vi "DynamicConstantCurrScan.vi"() -> ()   [LabVIEW 2014]
uses:
  <vilib>/userdefined/High Color/nirio_resource_hc.ctl
  <vilib>/Instr/_visa.llb/VISA Configure Serial Port (Instr).vi
  <vilib>/FPGAPlugInAG/PCIe-7851R/niLvFpga_Open_PCIe-7851R.vi
  <vilib>/rvi/interface/common/dynamic/niFpgaDynamicAddResources.vi
  <vilib>/Utility/error.llb/Error Cluster From Error Code.vi
  <vilib>/rvi/errors/niLvFpgaAdjustHostInterfaceError.vi
  <vilib>/FPGAPlugInAG/Dynamic/niLvFpga_Close_Dynamic.vi
  <vilib>/rvi/interface/nirviOpenFPGA/nirviOpenFPGA.xnode
  FPGA Bitfiles/FPGATest_FPGATarget_PIZApproaching_ngy2QjQf4ns.lvbitx
  <vilib>/rvi/interface/nirviReadWriteControl/nirviReadWriteControl.xnode
  <vilib>/rvi/interface/nirviCloseFPGA/nirviCloseFPGA.xnode
  FPGA Bitfiles/FPGATest_FPGATarget_ProbeAdjustment_Nyu9RVmYDZg.lvbitx
  FPGA Bitfiles/FPGATest_FPGATarget_PIZWithdraw_LXoQbY-wYvI.lvbitx
  NiFpgaLv.dll
  <vilib>/rvi/interface/Simulation/niFpgaSimulationCallBeginRW.vi
  NextXYPos.dll
panel:
  in  "zRisingLimitLen / um":dbl format="%#_13g"
  in  "ScanStop":bool
  out "refCurrIndex":i32
  out "preCurrIndexDia":i16(graph)
  out "ZPosDia":i16(graph)
  out "PIZPosIndex":i32
  out "preCurrIndex":i32
  in  "ApproachStop":bool
  out "ThresholdLowerBound":i32
  out "ThresholdUpperBound":i32
  in  "DeclineTolerantInterval %":dbl format="%#_13g"
  in  "AdjustStepMultiplier/0.305nm":i32
  in  "ApproachStepMultiplier/0.305nm":i32
  in  "PIZ":T1
  in  "ProbeBrokenIndex":i32
  in  "ThresholdIndex":i32
  in  "ScanNumToRefresh":i32
  out "YPos?":dbl
  out "XPos?":dbl
  in  "YInitStepLen / um":dbl format="%#_13g"
  in  "XInitStepLen / um":dbl format="%#_13g"
  in  "YDirTotalLen / um":dbl format="%#_13g"
  in  "XDirTotalLen / um":dbl format="%#_13g"
  in  "Y Init / um":dbl format="%#_13g"
  in  "X Init / um":dbl format="%#_13g"
  out "RoughXYZErr?":string
  in  "RoughXYZ":refnum<visa-resource-name>
  in  "AllLoopSleep ms":i32
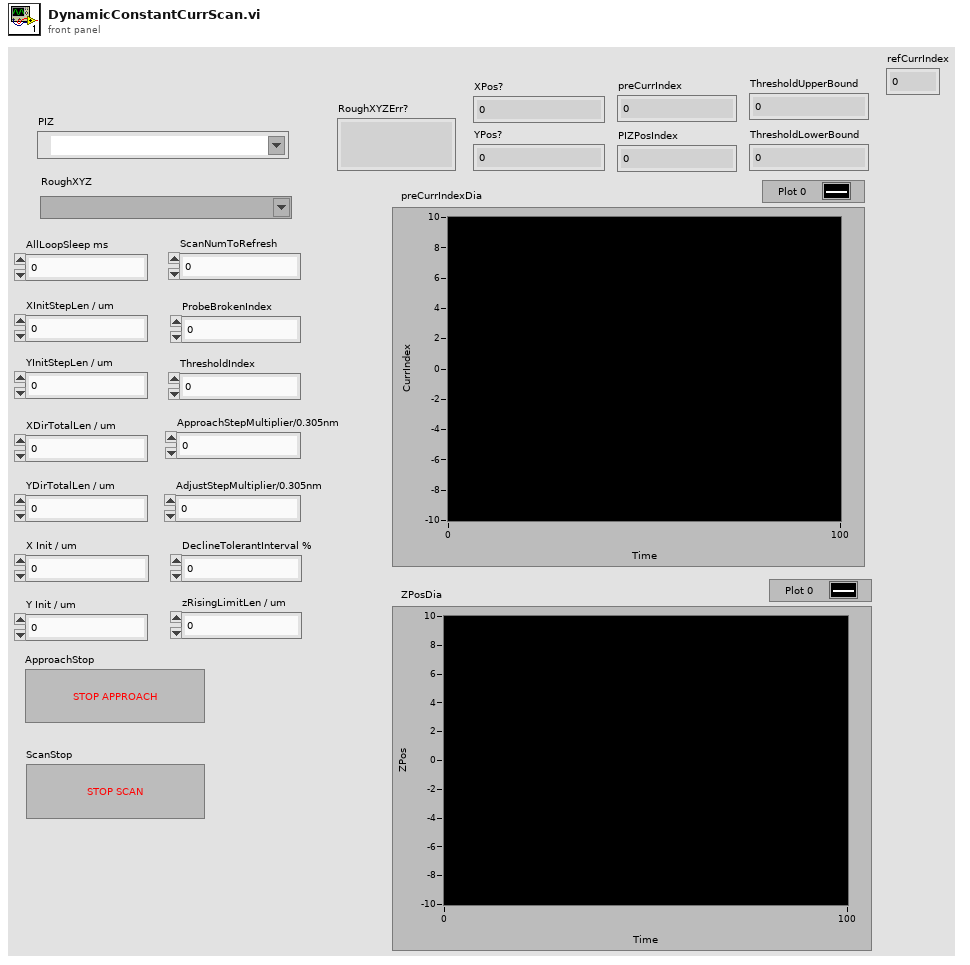
[diagram p1: front panel]
types:
  T1 = typedef "nirio_resource_hc.ctl" = tag
diagram:
  n1 = flat-sequence {
    tunnel: [w69] -> w52
    tunnel: [w68] -> w51
    tunnel: w52 -> [w111]
    tunnel: w51 -> [w110]
    tunnel: [w95] -> w50
    tunnel: [w94] -> w49
    tunnel: w50 -> [w113]
    tunnel: w49 -> [w112]
    tunnel: [w113] -> w48
    tunnel: [w112] -> w47
    tunnel: w48 -> [w118]
    tunnel: w47 -> [w117]
    tunnel: [w116] -> w46
    tunnel: [w115] -> w44
    tunnel: w46 -> [w144]
    tunnel: [w144] -> w45
    tunnel: w44 -> [w143]
    tunnel: [w143] -> w43
    tunnel: [w139] -> w42
    tunnel: [w138] -> w41
    tunnel: [w135] -> w40
    tunnel: w45 -> [w151]
    tunnel: w43 -> [w150]
    tunnel: w42 -> [w153]
    tunnel: w41 -> [w152]
    tunnel: w40 -> [w149]
    tunnel: [w146] -> w39
    tunnel: [w145] -> w38
    tunnel: w39 -> [w220]
    tunnel: w38 -> [w219]
    tunnel: [w220] -> w37
    tunnel: [w219] -> w36
    tunnel: [w214] -> w35
    tunnel: [w213] -> w34
    tunnel: [w213] -> w33
    tunnel: [1] -> w32
    tunnel: [w211] -> w31
    tunnel: [w210] -> w30
    tunnel: [w209] -> w29
    tunnel: [w208] -> w28
    tunnel: [0] -> w27
    tunnel: [w206] -> w26
    tunnel: [w206] -> w25
    tunnel: [w206] -> w24
    tunnel: [w206] -> w23
    tunnel: [i32[] []] -> w22
    tunnel: [w193] -> w21
    tunnel: [w192] -> w20
    tunnel: w37 -> [w248]
    tunnel: w36 -> [w247]
    tunnel: w35 -> [w246]
    tunnel: w34 -> [w237]
    tunnel: w33 -> [w236]
    tunnel: w32 -> [w240]
    tunnel: w31 -> [w239]
    tunnel: w30 -> [w238]
    tunnel: w29 -> [w242]
    tunnel: w28 -> [w241]
    tunnel: w27 -> [w243]
    tunnel: w26 -> [w230]
    tunnel: w25 -> [w229]
    tunnel: w24 -> [w228]
    tunnel: w23 -> [w227]
    tunnel: w22 -> [w226]
    tunnel: w21 -> [w245]
    tunnel: w20 -> [w244]
    tunnel: [w235] -> w19
    tunnel: [w234] -> w18
    tunnel: [w233] -> w17
    tunnel: [w232] -> w16
    tunnel: [w231] -> w15
    tunnel: [w225] -> w14
    tunnel: [w224] -> w13
    tunnel: [w223] -> w12
    tunnel: [w222] -> w11
    tunnel: w19 -> [_]
    tunnel: w18 -> [_]
    tunnel: w17 -> [_]
    tunnel: w16 -> [_]
    tunnel: w15 -> [_]
    tunnel: w14 -> [w863]
    tunnel: w13 -> [w861]
    tunnel: w12 -> [w860]
    tunnel: w11 -> [w862]
    tunnel: [w857] -> w10
    tunnel: [w856] -> w9
    tunnel: [w851] -> w8
    tunnel: [w850] -> w7
    tunnel: w10 -> [w869]
    tunnel: w9 -> [w868]
    tunnel: w8 -> [w871]
    tunnel: w7 -> [w870]
    tunnel: [w867] -> w6
    tunnel: [w866] -> w5
    tunnel: [w865] -> w4
    tunnel: [w864] -> w3
    tunnel: w6 -> [w906]
    tunnel: w5 -> [w905]
    tunnel: w4 -> [w904]
    tunnel: w3 -> [w903]
    tunnel: [w902] -> w2
    tunnel: [w901] -> w1
    tunnel: w2 -> [w915]
    tunnel: w1 -> [w914]
    frame #0 {
      n2 = call-poly "VISA Configure Serial Port"("VISA resource name"="RoughXYZ", "baud rate (9600)"=u32 115200) -> ("VISA resource name out"=w78:refnum<visa-resource-name>, "error out"=w77:errorcluster)  [unwired: 12 in]
      n3 = local write "DeclineTolerantInterval %"("DeclineTolerantInterval %") -> ()
      n4 = local write "AllLoopSleep ms"("AllLoopSleep ms") -> ()
      n5 = local write "XDirTotalLen / um"("XDirTotalLen / um") -> ()
      n6 = local write "YDirTotalLen / um"("YDirTotalLen / um") -> ()
      n7 = local write "XInitStepLen / um"("XInitStepLen / um") -> ()
      n8 = local write "YInitStepLen / um"("YInitStepLen / um") -> ()
      n9 = local write "zRisingLimitLen / um"("zRisingLimitLen / um") -> ()
      n10 = local write "X Init / um"("X Init / um") -> ()
      n11 = local write "Y Init / um"("Y Init / um") -> ()
      n12 = local write "PIZ"("PIZ") -> ()
      n13 = VISA Write(VISA resource name=w78, write buffer="ERR?\n", error in (no error)=w77) -> (VISA resource name out=w75:refnum<visa-resource-name>, error out=w74:errorcluster)  [unwired: 1 out]
      n14 = VISA Read(VISA resource name=w75, byte count=u32 128, error in (no error)=w74) -> (VISA resource name out=w72:refnum<visa-resource-name>, read buffer=→"RoughXYZErr?":string, error out=w71:errorcluster)  [unwired: 1 out]
      n15 = local write "ProbeBrokenIndex"("ProbeBrokenIndex") -> ()
      n16 = local write "ScanNumToRefresh"("ScanNumToRefresh") -> ()
      n17 = local write "ApproachStepMultiplier/0.305nm"("ApproachStepMultiplier/0.305nm") -> ()
      n18 = local write "ThresholdIndex"("ThresholdIndex") -> ()
      n19 = local write "AdjustStepMultiplier/0.305nm"("AdjustStepMultiplier/0.305nm") -> ()
      n20 = VISA Write(VISA resource name=w72, write buffer="ONL 1 1 2 1 3 1\nSVO A 1\nSVO B 1\nSVO C 1\nMOV A 0\nMOV B 0\n", error in (no error)=w71) -> (VISA resource name out=w69:refnum<visa-resource-name>, error out=w68:errorcluster)  [unwired: 1 out]
    }
    frame #1 {
      n21 = local read "DeclineTolerantInterval %"() -> (w92:dbl)
      n22 = local read "ThresholdIndex"() -> (w89:i32)
      n23 = local read "X Init / um"() -> (w107:dbl)
      n24 = Number To Fractional String(number=w107, precision (6)=i16 10) -> (F-format string=w105:string)  [unwired: 2 in]
      n25 = Concatenate Strings("MOV A " ("string"), w105, "\n" ("string")) -> (w102:string)
      n26 = Divide(x=w92, y=100.0) -> (x/y=w90:dbl)
      n27 = VISA Write(VISA resource name=w111, write buffer=w102, error in (no error)=w110) -> (VISA resource name out=w109:refnum<visa-resource-name>, error out=w108:errorcluster)  [unwired: 1 out]
      n28 = Multiply(x=w89, y=w90) -> (x*y=w88:dbl)
      n29 = local read "Y Init / um"() -> (w101:dbl)
      n30 = Add(x=w89, y=w88) -> (x+y=w87:dbl)
      n31 = Subtract(x=w89, y=w88) -> (x-y=w86:dbl)
      n32 = Round Toward +Infinity(x=w87) -> (ceil(x): smallest int >= x=w85:dbl)
      n33 = Wait (ms)(milliseconds to wait=u32 200) -> ()  [unwired: 1 out]
      n34 = Round Toward -Infinity(1:w86) -> (0:w84:dbl)
      n35 = To Long Integer(number=w85) -> (32bit integer=→"ThresholdUpperBound":i32)
      n36 = To Long Integer(number=w84) -> (32bit integer=→"ThresholdLowerBound":i32)
      n37 = Number To Fractional String(number=w101, precision (6)=i16 10) -> (F-format string=w98:string)  [unwired: 2 in]
      n38 = Concatenate Strings("MOV B " ("string"), w98, "\n" ("string")) -> (w96:string)
      n39 = VISA Write(VISA resource name=w109, write buffer=w96, error in (no error)=w108) -> (VISA resource name out=w95:refnum<visa-resource-name>, error out=w94:errorcluster)  [unwired: 1 out]
    }
    frame #2 {
      n40 = Wait (ms)(milliseconds to wait=u32 1500) -> ()  [unwired: 1 out]
    }
    frame #3 {
      n41 = VISA Write(VISA resource name=w118, write buffer="POS? A\n", error in (no error)=w117) -> (VISA resource name out=w133:refnum<visa-resource-name>, error out=w132:errorcluster)  [unwired: 1 out]
      n42 = VISA Read(VISA resource name=w133, byte count=u32 128, error in (no error)=w132) -> (VISA resource name out=w127:refnum<visa-resource-name>, read buffer=w124:string, error out=w126:errorcluster)  [unwired: 1 out]
      n43 = Fract/Exp String To Number(string=w124, offset=2) -> (number=→"XPos?":dbl)  [unwired: 2 in, 1 out]
      n44 = VISA Write(VISA resource name=w127, write buffer="POS? B\n", error in (no error)=w126) -> (VISA resource name out=w130:refnum<visa-resource-name>, error out=w129:errorcluster)  [unwired: 1 out]
      n45 = VISA Read(VISA resource name=w130, byte count=u32 128, error in (no error)=w129) -> (VISA resource name out=w116:refnum<visa-resource-name>, read buffer=w119:string, error out=w115:errorcluster)  [unwired: 1 out]
      n46 = Fract/Exp String To Number(string=w119, offset=2) -> (number=→"YPos?":dbl)  [unwired: 2 in, 1 out]
    }
    frame #4 {
      n47 = local read "PIZ"() -> (w142:T1)
      n48 = xnode "Open FPGA VI Reference"("resource name"=w142) -> ("FPGA VI Reference Out"=w141:refnum<k20>, "error out"=w140:errorcluster)  [unwired: 1 in]
      n49 = local read "ApproachStepMultiplier/0.305nm"() -> (w136:i32)
      n50 = local read "AllLoopSleep ms"() -> (w135:i32)
      n51 = local read "ThresholdIndex"() -> (w137:i32)
      n52 = xnode "Read/Write Control"("FPGA VI Reference In"=w141, "error in"=w140, "Sleep ms"=w135, "thresholdIndex"=w137, "stepMultiplier / 0.305nm"=w136) -> ("FPGA VI Reference Out"=w139:refnum<k20>, "error out"=w138:errorcluster)
    }
    frame #5 {
      n53 = while {
        tunnel: w153 -> [w172]
        tunnel: w152 -> [w171]
        tunnel: w151 -> [w166]
        tunnel: w150 -> [w164]
        tunnel: w149 -> [w160]
        tunnel: [w157] -> w148
        tunnel: [w156] -> w147
        tunnel: [w155] -> w146
        tunnel: [w154] -> w145
        stop <- w163 stop-if-true
        n54 = flat-sequence {
          tunnel: w172 -> [w184]
          tunnel: w171 -> [w183]
          tunnel: [w182] -> w170
          tunnel: [w181] -> w169
          tunnel: ["ApproachStop"] -> w168
          tunnel: [w179] -> w167
          tunnel: w166 -> [w179]
          tunnel: [w178] -> w165
          tunnel: w164 -> [w178]
          tunnel: [w177] -> w161
          tunnel: w160 -> [w177]
          tunnel: [w176] -> w159
          tunnel: w170 -> [w186]
          tunnel: w169 -> [w185]
          tunnel: [w191] -> w162
          tunnel: w168 -> [w191]
          tunnel: [w190] -> w155
          tunnel: w167 -> [w190]
          tunnel: w165 -> [w189]
          tunnel: [w189] -> w154
          tunnel: w161 -> [w188]
          tunnel: w159 -> [w187]
          tunnel: [w187] -> w158
          tunnel: [w186] -> w157
          tunnel: [w185] -> w156
          frame #0 {
            n55 = xnode "Read/Write Control"("FPGA VI Reference In"=w184, "error in"=w183, "stop"="ApproachStop") -> ("FPGA VI Reference Out"=w182:refnum<k20>, "error out"=w181:errorcluster, "preCurrIndex"=→"preCurrIndex" →"preCurrIndexDia":i16, "PIZPos"=→"PIZPosIndex" →"ZPosDia":i16, "Approached?"=w176:bool, "refCurrIndex"=→"refCurrIndex":i16)
          }
          frame #1 {
            n56 = Wait (ms)(milliseconds to wait=w188) -> ()  [unwired: 1 out]
          }
        }
        n57 = Or(x=w158, y=w162) -> (x .or. y?=w163:bool)
      }
      n58 = xnode "Close FPGA VI Reference"("FPGA VI Reference In"=w148, "error in"=w147) -> ()  [unwired: 1 out]
    }
    frame #6 {
      w206 = dbl[] []
      w213 = 0
      # "zPosIndex"
      # "yReal"
      # "yCal"
      # "xReal"
      # "xCal"
      # "LastZPos"
      # "yCalPos"
      # "xCalPos"
      # "yStepLen"
      # "xStepLen"
      # "xVel"
      # "yCounting"
      # "xCounting"
      # "xPreviousNum"
      n59 = local read "PIZ"() -> (w204:T1)
      n60 = local read "XDirTotalLen / um"() -> (w218:dbl)
      n61 = local read "XInitStepLen / um"() -> (w217:dbl)
      n62 = Wait (ms)(milliseconds to wait=u32 50) -> ()  [unwired: 1 out]
      n63 = xnode "Open FPGA VI Reference"("resource name"=w204) -> ("FPGA VI Reference Out"=w203:refnum<k20>, "error out"=w202:errorcluster)  [unwired: 1 in]
      n64 = local read "AdjustStepMultiplier/0.305nm"() -> (w196:i32)
      n65 = local read "ThresholdUpperBound"() -> (w201:i32)
      n66 = local read "ThresholdLowerBound"() -> (w200:i32)
      n67 = local read "ScanNumToRefresh"() -> (w197:i32)
      n68 = local read "ProbeBrokenIndex"() -> (w198:i32)
      n69 = local read "AllLoopSleep ms"() -> (w194:i32)
      n70 = local read "ThresholdIndex"() -> (w199:i32)
      n71 = local read "refCurrIndex"() -> (w195:i32)
      n72 = Divide(x=w218, y=w217) -> (x/y=w216:dbl)
      n73 = Round Toward +Infinity(x=w216) -> (ceil(x): smallest int >= x=w215:dbl)
      n74 = To Long Integer(number=w215) -> (32bit integer=w214:i32)
      n75 = xnode "Read/Write Control"("FPGA VI Reference In"=w203, "error in"=w202, "ThresholdUpperBound"=w201, "ThresholdLowerBound"=w200, "ThresholdIndex"=w199, "ProbeBrokenIndex"=w198, "ScanNumToRefresh"=w197, "stepMultiplier/0.305nm"=w196, "refCurrIndex"=w195, "Sleep ms"=w194) -> ("FPGA VI Reference Out"=w193:refnum<k20>, "error out"=w192:errorcluster)
      n76 = local read "XInitStepLen / um"() -> (w211:dbl)
      n77 = local read "YInitStepLen / um"() -> (w210:dbl)
      n78 = local read "X Init / um"() -> (w209:dbl)
      n79 = local read "Y Init / um"() -> (w208:dbl)
    }
    frame #7 {
      n80 = while {
        tunnel: w248 -> [w405]
        tunnel: w247 -> [w404]
        tunnel: w246 -> [w365]
        tunnel: w245 -> [w393]
        tunnel: w244 -> [w392]
        shift-right: [w285] -> _
        shift-left: w237 -> [w274]
        shift-right: [w284] -> _
        shift-left: w236 -> [w273]
        shift-right: [w283] -> _
        shift-left: w240 -> [w277]
        shift-right: [w281] -> _
        shift-left: w239 -> [w276]
        shift-right: [w282] -> _
        shift-left: w238 -> [w275]
        shift-right: [w288] -> _
        shift-left: w242 -> [w279]
        shift-right: [w287] -> _
        shift-left: w241 -> [w278]
        shift-right: [w286] -> _
        shift-left: w243 -> [w280]
        shift-right: [w272] -> w235
        shift-left: w230 -> [w267]
        shift-right: [w271] -> w234
        shift-left: w229 -> [w266]
        shift-right: [w270] -> w233
        shift-left: w228 -> [w265]
        shift-right: [w269] -> w232
        shift-left: w227 -> [w264]
        shift-right: [w268] -> w231
        shift-left: w226 -> [w263]
        tunnel: [w262] -> w224
        tunnel: [w261] -> w223
        tunnel: [w258] -> w225
        tunnel: [w257] -> w222
        stop <- w253 stop-if-true
        n81 = flat-sequence {
          tunnel: w405 -> [w441]
          tunnel: w404 -> [w440]
          tunnel: [w429] -> w403
          tunnel: [w428] -> w402
          tunnel: [w421] -> w401
          tunnel: w279 -> [w421]
          tunnel: [w420] -> w400
          tunnel: w278 -> [w420]
          tunnel: [w419] -> w399
          tunnel: w280 -> [w419]
          tunnel: w393 -> [w418]
          tunnel: w392 -> [w417]
          tunnel: [w418] -> w389
          tunnel: [w417] -> w386
          tunnel: [w416] -> w380
          tunnel: w267 -> [w416]
          tunnel: [w415] -> w379
          tunnel: w266 -> [w415]
          tunnel: [w414] -> w378
          tunnel: w265 -> [w414]
          tunnel: [w413] -> w377
          tunnel: w264 -> [w413]
          tunnel: [w412] -> w374
          tunnel: w263 -> [w412]
          tunnel: [w411] -> w369
          tunnel: w274 -> [w411]
          tunnel: [w410] -> w368
          tunnel: w273 -> [w410]
          tunnel: [w409] -> w366
          tunnel: w365 -> [w409]
          tunnel: [w408] -> w363
          tunnel: w277 -> [w408]
          tunnel: [w407] -> w361
          tunnel: w276 -> [w407]
          tunnel: [w406] -> w360
          tunnel: w275 -> [w406]
          tunnel: w403 -> [w473]
          tunnel: w402 -> [w472]
          tunnel: w401 -> [w463]
          tunnel: w400 -> [w458]
          tunnel: w399 -> [w457]
          tunnel: [w463] -> w398
          tunnel: [w458] -> w397
          tunnel: [w457] -> w396
          tunnel: [w456] -> w395
          tunnel: [w455] -> w394
          tunnel: [w454] -> w390
          tunnel: w389 -> [w454]
          tunnel: [w453] -> w387
          tunnel: w386 -> [w453]
          tunnel: w380 -> [w452]
          tunnel: w379 -> [w451]
          tunnel: w378 -> [w450]
          tunnel: w377 -> [w449]
          tunnel: [w452] -> w376
          tunnel: [w451] -> w375
          tunnel: w374 -> [w448]
          tunnel: [w450] -> w373
          tunnel: [w449] -> w372
          tunnel: [w448] -> w371
          tunnel: [w447] -> w370
          tunnel: w369 -> [w447]
          tunnel: w368 -> [w446]
          tunnel: [w446] -> w367
          tunnel: w366 -> [w445]
          tunnel: [w445] -> w364
          tunnel: w363 -> [w444]
          tunnel: [w444] -> w362
          tunnel: w361 -> [w443]
          tunnel: w360 -> [w442]
          tunnel: [w443] -> w359
          tunnel: [w442] -> w358
          tunnel: w398 -> [w487]
          tunnel: w397 -> [w486]
          tunnel: w396 -> [w485]
          tunnel: w395 -> [w489]
          tunnel: w394 -> [w488]
          tunnel: [w491] -> w391
          tunnel: w390 -> [w491]
          tunnel: [w490] -> w388
          tunnel: w387 -> [w490]
          tunnel: [w489] -> w385
          tunnel: [w488] -> w384
          tunnel: [w487] -> w383
          tunnel: [w486] -> w382
          tunnel: [w485] -> w381
          tunnel: w376 -> [w484]
          tunnel: w375 -> [w483]
          tunnel: w373 -> [w482]
          tunnel: w372 -> [w481]
          tunnel: w371 -> [w480]
          tunnel: w370 -> [w479]
          tunnel: w367 -> [w478]
          tunnel: w364 -> [w477]
          tunnel: w362 -> [w476]
          tunnel: w359 -> [w475]
          tunnel: w358 -> [w474]
          tunnel: [w484] -> w357
          tunnel: [w483] -> w356
          tunnel: [w482] -> w355
          tunnel: [w481] -> w354
          tunnel: [w480] -> w353
          tunnel: [w479] -> w352
          tunnel: [w478] -> w351
          tunnel: [w477] -> w350
          tunnel: [w476] -> w349
          tunnel: [w475] -> w348
          tunnel: [w474] -> w347
          tunnel: w391 -> [w531]
          tunnel: w388 -> [w530]
          tunnel: w385 -> [w529]
          tunnel: w384 -> [w528]
          tunnel: w383 -> [w514]
          tunnel: w382 -> [w515]
          tunnel: w381 -> [w516]
          tunnel: w357 -> [w527]
          tunnel: w356 -> [w526]
          tunnel: w355 -> [w525]
          tunnel: w354 -> [w524]
          tunnel: w353 -> [w523]
          tunnel: w352 -> [w522]
          tunnel: w351 -> [w521]
          tunnel: w350 -> [w520]
          tunnel: w349 -> [w519]
          tunnel: w348 -> [w518]
          tunnel: w347 -> [w517]
          tunnel: [w513] -> w346
          tunnel: [w512] -> w345
          tunnel: [w511] -> w344
          tunnel: [w510] -> w343
          tunnel: [w509] -> w342
          tunnel: [w508] -> w341
          tunnel: [w507] -> w340
          tunnel: [w506] -> w339
          tunnel: [w505] -> w338
          tunnel: [w504] -> w337
          tunnel: [w503] -> w336
          tunnel: [w502] -> w335
          tunnel: [w501] -> w334
          tunnel: [w500] -> w333
          tunnel: [w499] -> w332
          tunnel: [w498] -> w331
          tunnel: [w497] -> w330
          tunnel: [w496] -> w329
          tunnel: [w495] -> w328
          tunnel: [w494] -> w297
          tunnel: [w493] -> w252
          tunnel: w346 -> [w724]
          tunnel: w345 -> [w723]
          tunnel: w344 -> [w736]
          tunnel: w343 -> [w735]
          tunnel: w342 -> [w734]
          tunnel: w341 -> [w733]
          tunnel: w340 -> [w732]
          tunnel: w339 -> [w731]
          tunnel: w338 -> [w730]
          tunnel: w337 -> [w729]
          tunnel: w336 -> [w728]
          tunnel: w335 -> [w727]
          tunnel: w334 -> [w726]
          tunnel: w333 -> [w725]
          tunnel: w332 -> [w744]
          tunnel: w331 -> [w743]
          tunnel: w330 -> [w740]
          tunnel: w329 -> [w739]
          tunnel: w328 -> [w745]
          tunnel: [w742] -> w327
          tunnel: [w741] -> w326
          tunnel: [w738] -> w325
          tunnel: [w737] -> w324
          tunnel: [w736] -> w323
          tunnel: [w735] -> w322
          tunnel: [w734] -> w321
          tunnel: [w733] -> w320
          tunnel: [w732] -> w319
          tunnel: [w731] -> w318
          tunnel: [w730] -> w317
          tunnel: [w729] -> w316
          tunnel: [w728] -> w315
          tunnel: [w727] -> w314
          tunnel: [w726] -> w313
          tunnel: [w725] -> w312
          tunnel: w297 -> [w722]
          tunnel: [w724] -> w296
          tunnel: [w723] -> w295
          tunnel: [w722] -> w294
          tunnel: w252 -> [w721]
          tunnel: [w721] -> w251
          tunnel: w327 -> [w810]
          tunnel: w326 -> [w809]
          tunnel: w325 -> [w793]
          tunnel: w324 -> [w792]
          tunnel: w323 -> [w808]
          tunnel: w322 -> [w807]
          tunnel: w321 -> [w806]
          tunnel: w320 -> [w805]
          tunnel: w319 -> [w804]
          tunnel: w318 -> [w803]
          tunnel: w317 -> [w802]
          tunnel: w316 -> [w801]
          tunnel: w315 -> [w800]
          tunnel: w314 -> [w799]
          tunnel: w313 -> [w798]
          tunnel: w312 -> [w797]
          tunnel: [w810] -> w311
          tunnel: [w809] -> w310
          tunnel: [w808] -> w309
          tunnel: [w807] -> w308
          tunnel: [w806] -> w307
          tunnel: [w805] -> w306
          tunnel: [w804] -> w305
          tunnel: [w803] -> w304
          tunnel: [w802] -> w303
          tunnel: [w801] -> w302
          tunnel: [w800] -> w301
          tunnel: [w799] -> w300
          tunnel: [w798] -> w299
          tunnel: [w797] -> w298
          tunnel: w296 -> [w796]
          tunnel: w295 -> [w795]
          tunnel: w294 -> [w794]
          tunnel: [w796] -> w293
          tunnel: [w795] -> w292
          tunnel: [w794] -> w291
          tunnel: [w793] -> w290
          tunnel: [w792] -> w289
          tunnel: w251 -> [w791]
          tunnel: [w791] -> w250
          tunnel: w291 -> [w827]
          tunnel: w292 -> [w835]
          tunnel: w293 -> [w837]
          tunnel: w298 -> [w823]
          tunnel: w299 -> [w825]
          tunnel: w300 -> [w829]
          tunnel: w301 -> [w844]
          tunnel: w302 -> [w831]
          tunnel: w303 -> [w833]
          tunnel: w304 -> [w842]
          tunnel: w305 -> [w817]
          tunnel: w306 -> [w818]
          tunnel: w307 -> [w819]
          tunnel: w308 -> [w820]
          tunnel: w309 -> [w821]
          tunnel: w310 -> [w813]
          tunnel: w311 -> [w814]
          tunnel: w290 -> [w816]
          tunnel: w289 -> [w815]
          tunnel: [w838] -> w256
          tunnel: [w836] -> w288
          tunnel: [w834] -> w287
          tunnel: [w826] -> w286
          tunnel: [w832] -> w285
          tunnel: [w830] -> w284
          tunnel: [w828] -> w283
          tunnel: [w824] -> w281
          tunnel: [w822] -> w282
          tunnel: [w821] -> w272
          tunnel: [w820] -> w271
          tunnel: [w819] -> w270
          tunnel: [w818] -> w269
          tunnel: [w817] -> w268
          tunnel: [w816] -> w262
          tunnel: [w815] -> w261
          tunnel: [w814] -> w260
          tunnel: [w813] -> w259
          tunnel: w250 -> [w812]
          tunnel: [w812] -> w249
          frame #0 {
            n82 = VISA Write(VISA resource name=w441, write buffer="POS? A\n", error in (no error)=w440) -> (VISA resource name out=w438:refnum<visa-resource-name>, error out=w437:errorcluster)  [unwired: 1 out]
            n83 = VISA Read(VISA resource name=w438, byte count=u32 128, error in (no error)=w437) -> (VISA resource name out=w431:refnum<visa-resource-name>, read buffer=w427:string, error out=w430:errorcluster)  [unwired: 1 out]
            n84 = Fract/Exp String To Number(string=w427, offset=2) -> (number=w423:dbl)  [unwired: 2 in, 1 out]
            n85 = local write "XPos?"(w423) -> ()
            n86 = VISA Write(VISA resource name=w431, write buffer="POS? B\n", error in (no error)=w430) -> (VISA resource name out=w434:refnum<visa-resource-name>, error out=w433:errorcluster)  [unwired: 1 out]
            n87 = VISA Read(VISA resource name=w434, byte count=u32 128, error in (no error)=w433) -> (VISA resource name out=w429:refnum<visa-resource-name>, read buffer=w425:string, error out=w428:errorcluster)  [unwired: 1 out]
            n88 = Fract/Exp String To Number(string=w425, offset=2) -> (number=w422:dbl)  [unwired: 2 in, 1 out]
            n89 = local write "YPos?"(w422) -> ()
          }
          frame #1 {
            n90 = Number To Fractional String(number=w463, precision (6)=i16 10) -> (F-format string=w465:string)  [unwired: 2 in]
            n91 = Concatenate Strings("MOV A " ("string"), w465, "\n" ("string")) -> (w469:string)
            n92 = VISA Write(VISA resource name=w473, write buffer=w469, error in (no error)=w472) -> (VISA resource name out=w471:refnum<visa-resource-name>, error out=w470:errorcluster)  [unwired: 1 out]
            n93 = Number To Fractional String(number=w458, precision (6)=i16 10) -> (F-format string=w459:string)  [unwired: 2 in]
            n94 = Concatenate Strings("MOV B " ("string"), w459, "\n" ("string")) -> (w468:string)
            n95 = VISA Write(VISA resource name=w471, write buffer=w468, error in (no error)=w470) -> (VISA resource name out=w456:refnum<visa-resource-name>, error out=w455:errorcluster)  [unwired: 1 out]
          }
          frame #2 {
            n96 = Wait (ms)(milliseconds to wait=u32 1) -> ()  [unwired: 1 out]
          }
          frame #3 {
            n97 = while {
              tunnel: w531 -> [w585]
              tunnel: w530 -> [w584]
              tunnel: w529 -> [w583]
              tunnel: w528 -> [w582]
              tunnel: w527 -> [w596]
              tunnel: w526 -> [w595]
              tunnel: w525 -> [w594]
              tunnel: w524 -> [w593]
              tunnel: w523 -> [w592]
              tunnel: w522 -> [w591]
              tunnel: w521 -> [w590]
              tunnel: w520 -> [w589]
              tunnel: w519 -> [w588]
              tunnel: w518 -> [w587]
              tunnel: w517 -> [w586]
              tunnel: w516 -> [w562]
              tunnel: w515 -> [w563]
              tunnel: w514 -> [w564]
              tunnel: [w558] -> w513
              tunnel: [w557] -> w512
              tunnel: [w551] -> w511
              tunnel: [w550] -> w510
              tunnel: [w549] -> w509
              tunnel: [w548] -> w508
              tunnel: [w547] -> w507
              tunnel: [w546] -> w506
              tunnel: [w545] -> w505
              tunnel: [w544] -> w504
              tunnel: [w543] -> w503
              tunnel: [w542] -> w502
              tunnel: [w541] -> w501
              tunnel: [w540] -> w500
              tunnel: [w539] -> w499
              tunnel: [w538] -> w498
              tunnel: [w537] -> w497
              tunnel: [w536] -> w496
              tunnel: [w535] -> w495
              tunnel: [w533] -> w494
              tunnel: [w532] -> w493
              stop <- w553 stop-if-true
              n98 = flat-sequence {
                tunnel: w596 -> [w606]
                tunnel: w595 -> [w607]
                tunnel: w594 -> [w608]
                tunnel: w593 -> [w609]
                tunnel: w592 -> [w610]
                tunnel: w591 -> [w611]
                tunnel: w590 -> [w612]
                tunnel: w589 -> [w613]
                tunnel: w588 -> [w614]
                tunnel: w587 -> [w615]
                tunnel: w586 -> [w616]
                tunnel: w585 -> [w622]
                tunnel: w584 -> [w621]
                tunnel: w583 -> [w605]
                tunnel: w582 -> [w604]
                tunnel: [w620] -> w581
                tunnel: [w619] -> w580
                tunnel: [w618] -> w579
                tunnel: [w617] -> w578
                tunnel: [w616] -> w577
                tunnel: [w615] -> w576
                tunnel: [w614] -> w575
                tunnel: [w613] -> w574
                tunnel: [w612] -> w573
                tunnel: [w611] -> w572
                tunnel: [w610] -> w571
                tunnel: [w609] -> w570
                tunnel: [w608] -> w569
                tunnel: [w607] -> w568
                tunnel: [w606] -> w567
                tunnel: [w605] -> w566
                tunnel: [w604] -> w565
                tunnel: w564 -> [w602]
                tunnel: w563 -> [w601]
                tunnel: w562 -> [w603]
                tunnel: [w603] -> w561
                tunnel: [w602] -> w560
                tunnel: [w601] -> w559
                tunnel: [w602] -> w556
                tunnel: [w601] -> w555
                tunnel: ["ScanStop"] -> w554
                tunnel: [w599] -> w552
                tunnel: [w598] -> w534
                tunnel: w581 -> [w663]
                tunnel: w580 -> [w662]
                tunnel: w579 -> [w647]
                tunnel: [w661] -> w539
                tunnel: [w660] -> w538
                tunnel: w578 -> [w659]
                tunnel: w577 -> [w653]
                tunnel: w576 -> [w654]
                tunnel: w575 -> [w655]
                tunnel: w574 -> [w656]
                tunnel: w573 -> [w657]
                tunnel: w572 -> [w658]
                tunnel: w571 -> [w652]
                tunnel: w570 -> [w651]
                tunnel: w569 -> [w650]
                tunnel: w568 -> [w649]
                tunnel: w567 -> [w648]
                tunnel: w566 -> [w634]
                tunnel: w565 -> [w633]
                tunnel: [w646] -> w546
                tunnel: w561 -> [w623]
                tunnel: w560 -> [w645]
                tunnel: w559 -> [w644]
                tunnel: [w645] -> w558
                tunnel: [w644] -> w557
                tunnel: w556 -> [w643]
                tunnel: w555 -> [w642]
                tunnel: [w641] -> w532
                tunnel: w554 -> [w641]
                tunnel: [w640] -> w535
                tunnel: w552 -> [w640]
                tunnel: [w639] -> w547
                tunnel: [w638] -> w548
                tunnel: [w637] -> w549
                tunnel: [w636] -> w550
                tunnel: [w635] -> w551
                tunnel: [w632] -> w545
                tunnel: [w631] -> w544
                tunnel: [w630] -> w543
                tunnel: [w629] -> w542
                tunnel: [w628] -> w541
                tunnel: [w627] -> w540
                tunnel: [w626] -> w537
                tunnel: [w625] -> w536
                tunnel: w534 -> [w624]
                tunnel: [w623] -> w533
                frame #0 {
                  n99 = xnode "Read/Write Control"("FPGA VI Reference In"=w622, "error in"=w621, "stop"="ScanStop") -> ("FPGA VI Reference Out"=w620:refnum<k20>, "error out"=w619:errorcluster, "InPlace?"=w617:bool, "Reversing?"=w599:bool, "PIZPos"=w618:i16, "preCurrIndex"=w597:i16)
                  n100 = local write "ZPosDia"(w597) -> ()
                  n101 = local write "preCurrIndex"(w597) -> ()
                  n102 = local read "AllLoopSleep ms"() -> (w598:i32)
                }
                frame #1 {
                  n103 = Wait (ms)(milliseconds to wait=w624) -> ()  [unwired: 1 out]
                  n104 = case shown="True" w659 {
                    tunnel: w663 -> [w679 w720]
                    tunnel: w662 -> [w678 w719]
                    tunnel: [w679 w720] -> w661
                    tunnel: [w678 w719] -> w660
                    tunnel: w658 -> [w671 w687]
                    tunnel: w657 -> [w670 w686]
                    tunnel: w656 -> [w669 w685]
                    tunnel: w655 -> [w668 w684]
                    tunnel: w654 -> [w667 w683]
                    tunnel: w653 -> [w666 w682]
                    tunnel: w652 -> [w672 w709]
                    tunnel: w651 -> [w673 w712]
                    tunnel: w650 -> [w674 w714]
                    tunnel: w649 -> [w675 w716]
                    tunnel: w648 -> [w676 w718]
                    tunnel: w647 -> [_ w708]
                    tunnel: [w677 w708] -> w646
                    tunnel: w623 -> [w677 _]
                    tunnel: w643 -> [_ w707]
                    tunnel: w642 -> [_ w706]
                    tunnel: [w676 w717] -> w635
                    tunnel: [w675 w715] -> w636
                    tunnel: [w674 w713] -> w637
                    tunnel: [w673 w711] -> w638
                    tunnel: [w672 w710] -> w639
                    tunnel: w634 -> [w665 w695]
                    tunnel: w633 -> [w664 w694]
                    tunnel: [w665 w689] -> w626
                    tunnel: [w664 w688] -> w625
                    tunnel: [w671 w687] -> w632
                    tunnel: [w670 w686] -> w631
                    tunnel: [w669 w685] -> w630
                    tunnel: [w668 w684] -> w629
                    tunnel: [w667 w683] -> w628
                    tunnel: [w666 w682] -> w627
                    frame False {
                    }
                    frame True {
                      # "PIZPrePos"
                      n105 = Build Array (concatenate)(w718, w707) -> (w717:dbl[])
                      n106 = VISA Write(VISA resource name=w695, write buffer="POS? A\n", error in (no error)=w694) -> (VISA resource name out=w704:refnum<visa-resource-name>, error out=w703:errorcluster)  [unwired: 1 out]
                      n107 = VISA Read(VISA resource name=w704, byte count=u32 128, error in (no error)=w703) -> (VISA resource name out=w697:refnum<visa-resource-name>, read buffer=w692:string, error out=w696:errorcluster)  [unwired: 1 out]
                      n108 = Fract/Exp String To Number(string=w692, offset=2) -> (number=w681:dbl)  [unwired: 2 in, 1 out]
                      n109 = Build Array (concatenate)(w716, w681) -> (w715:dbl[])
                      n110 = local write "XPos?"(w681) -> ()
                      n111 = VISA Write(VISA resource name=w697, write buffer="POS? B\n", error in (no error)=w696) -> (VISA resource name out=w700:refnum<visa-resource-name>, error out=w699:errorcluster)  [unwired: 1 out]
                      n112 = Build Array (concatenate)(w714, w706) -> (w713:dbl[])
                      n113 = VISA Read(VISA resource name=w700, byte count=u32 128, error in (no error)=w699) -> (VISA resource name out=w689:refnum<visa-resource-name>, read buffer=w693:string, error out=w688:errorcluster)  [unwired: 1 out]
                      n114 = Fract/Exp String To Number(string=w693, offset=2) -> (number=w680:dbl)  [unwired: 2 in, 1 out]
                      n115 = Build Array (concatenate)(w712, w680) -> (w711:dbl[])
                      n116 = local write "YPos?"(w680) -> ()
                      n117 = Build Array (concatenate)(w709, w708) -> (w710:i32[])
                    }
                  }
                }
              }
              n118 = Or(x=w532, y=w535) -> (x .or. y?=w553:bool)
            }
          }
          frame #4 {
            n119 = case shown="True" w745 {
              tunnel: w744 -> [w749 w756]
              tunnel: w743 -> [w748 w755]
              tunnel: [w749 w752] -> w742
              tunnel: [w748 w751] -> w741
              tunnel: w740 -> [w747 w758]
              tunnel: w739 -> [w746 w757]
              tunnel: [w747 w754] -> w738
              tunnel: [w746 w753] -> w737
              frame False {
              }
              frame True {
                n120 = while {
                  tunnel: w758 -> [w772]
                  tunnel: w757 -> [w771]
                  tunnel: w756 -> [w774]
                  tunnel: w755 -> [w773]
                  tunnel: [w768] -> w754
                  tunnel: [w767] -> w753
                  tunnel: [w764] -> w752
                  tunnel: [w763] -> w751
                  tunnel: [w761] -> w750
                  stop <- w759 stop-if-true
                  n121 = flat-sequence {
                    tunnel: w774 -> [w781]
                    tunnel: w773 -> [w780]
                    tunnel: w772 -> [w783]
                    tunnel: w771 -> [w782]
                    tunnel: [w783] -> w770
                    tunnel: [w782] -> w769
                    tunnel: [w779] -> w766
                    tunnel: [w778] -> w765
                    tunnel: [w777] -> w762
                    tunnel: [w776] -> w760
                    tunnel: w770 -> [w790]
                    tunnel: w769 -> [w789]
                    tunnel: [w790] -> w768
                    tunnel: [w789] -> w767
                    tunnel: w766 -> [w787]
                    tunnel: w765 -> [w786]
                    tunnel: [w787] -> w764
                    tunnel: [w786] -> w763
                    tunnel: [w785] -> w761
                    tunnel: w762 -> [w785]
                    tunnel: w760 -> [w784]
                    tunnel: [w784] -> w759
                    frame #0 {
                      n122 = xnode "Read/Write Control"("FPGA VI Reference In"=w781, "error in"=w780) -> ("FPGA VI Reference Out"=w779:refnum<k20>, "error out"=w778:errorcluster, "Approached?"=w776:bool, "PIZPos"=w775:i16, "NewRefCurrIndex"=w777:i16)
                      n123 = local write "PIZPosIndex"(w775) -> ()
                      n124 = local write "ZPosDia"(w775) -> ()
                    }
                    frame #1 {
                      n125 = local read "AllLoopSleep ms"() -> (w788:i32)
                      n126 = Wait (ms)(milliseconds to wait=w788) -> ()  [unwired: 1 out]
                    }
                  }
                }
                n127 = local write "refCurrIndex"(w750) -> ()
              }
            }
          }
          frame #5 {
            # "zPosIndex"
            # "yReal"
            # "yCal"
            # "xReal"
            # "xCal"
            # "PIZPrePos"
            # "xCounting"
            # "yCounting"
            # "xPreviousNum"
            # "xVel"
            # "xStepLen"
            # "yStepLen"
            # "LastZPos"
            # "yCalPos"
            # "xCalPos"
            n128 = Wait (ms)(milliseconds to wait=u32 1) -> ()  [unwired: 1 out]
          }
          frame #6 {
            n129 = local read "zRisingLimitLen / um"() -> (w839:dbl)
            n130 = local read "XDirTotalLen / um"() -> (w849:dbl)
            n131 = local read "YDirTotalLen / um"() -> (w848:dbl)
            n132 = local read "XInitStepLen / um"() -> (w841:dbl)
            n133 = local read "YInitStepLen / um"() -> (w840:dbl)
            n134 = local read "X Init / um"() -> (w843:dbl)
            n135 = local read "Y Init / um"() -> (w847:dbl)
            n136 = Add(x=w849, y=w843) -> (x+y=w846:dbl)
            n137 = Add(x=w848, y=w847) -> (x+y=w845:dbl)
            n138 = dll-call lib="C:/Users/Liu Chongyang/Desktop/Hopping_WangYunong/NextXYPos.dll" fn="?ModifyNextPos@@YAHNNNHPAN0PAH11HH00NNN@Z"("xMaxMov"=w846, "yMaxMov"=w845, "xInitPt"=w843, "xPreviousNum"=w844, "calXpos"=w837, "calYPos"=w835, "xCounting"=w833, "yCounting"=w831, "xVel"=w829, "lastZPos"=w827, "preZPos"=w842, "xStepLen"=w825, "yStepLen"=w823, "xInitStepLen"=w841, "yInitStepLen"=w840, "zRisingLimitLen"=w839) -> ("return type"=w838:i32, "calXpos"=w836:dbl, "calYPos"=w834:dbl, "xCounting"=w832:i32, "yCounting"=w830:i32, "xVel"=w828:i32, "preZPos"=w826:i32, "xStepLen"=w824:dbl, "yStepLen"=w822:dbl)  [unwired: 11 in, 2 out]
          }
        }
        n139 = Equal?(x=w256, y=1) -> (x = y?=w254:bool)
        n140 = Or(x=w254, y=w249) -> (x .or. y?=w253:bool)
        n141 = xnode "Read/Write Control"("FPGA VI Reference In"=w260, "error in"=w259, "Terminal"=w253) -> ("FPGA VI Reference Out"=w258:refnum<k20>, "error out"=w257:errorcluster)
      }
    }
    frame #8 {
      n142 = xnode "Close FPGA VI Reference"("FPGA VI Reference In"=w863, "error in"=w862) -> ()  [unwired: 1 out]
      n143 = local read "PIZ"() -> (w855:T1)
      n144 = VISA Write(VISA resource name=w861, write buffer="MOV C 0\n", error in (no error)=w860) -> (VISA resource name out=w857:refnum<visa-resource-name>, error out=w856:errorcluster)  [unwired: 1 out]
      n145 = xnode "Open FPGA VI Reference"("resource name"=w855) -> ("FPGA VI Reference Out"=w854:refnum<k20>, "error out"=w853:errorcluster)  [unwired: 1 in]
      n146 = Wait (ms)(milliseconds to wait=u32 50) -> ()  [unwired: 1 out]
      n147 = local read "AllLoopSleep ms"() -> (w852:i32)
      n148 = xnode "Read/Write Control"("FPGA VI Reference In"=w854, "error in"=w853, "Sleep ms"=w852) -> ("FPGA VI Reference Out"=w851:refnum<k20>, "error out"=w850:errorcluster)
    }
    frame #9 {
      n149 = while {
        tunnel: w871 -> [w885]
        tunnel: w870 -> [w884]
        tunnel: w869 -> [w883]
        tunnel: w868 -> [w882]
        tunnel: [w875] -> w867
        tunnel: [w874] -> w866
        tunnel: [w873] -> w865
        tunnel: [w872] -> w864
        stop <- w879 stop-if-true
        n150 = flat-sequence {
          tunnel: w885 -> [w892]
          tunnel: w884 -> [w891]
          tunnel: w883 -> [w894]
          tunnel: w882 -> [w893]
          tunnel: [w894] -> w881
          tunnel: [w893] -> w880
          tunnel: [w890] -> w878
          tunnel: [w889] -> w877
          tunnel: [w888] -> w876
          tunnel: w881 -> [w899]
          tunnel: w880 -> [w898]
          tunnel: [w899] -> w873
          tunnel: [w898] -> w872
          tunnel: [w897] -> w879
          tunnel: w878 -> [w897]
          tunnel: w877 -> [w896]
          tunnel: w876 -> [w895]
          tunnel: [w896] -> w875
          tunnel: [w895] -> w874
          frame #0 {
            n151 = xnode "Read/Write Control"("FPGA VI Reference In"=w892, "error in"=w891) -> ("FPGA VI Reference Out"=w889:refnum<k20>, "error out"=w888:errorcluster, "PIZPos?"=w887:i16, "preCurrIndex"=w886:i16, "Withdrawn?"=w890:bool)
            n152 = local write "preCurrIndex"(w886) -> ()
            n153 = local write "preCurrIndexDia"(w886) -> ()
            n154 = local write "PIZPosIndex"(w887) -> ()
            n155 = local write "ZPosDia"(w887) -> ()
          }
          frame #1 {
          }
        }
      }
    }
    frame #10 {
      n156 = xnode "Close FPGA VI Reference"("FPGA VI Reference In"=w906, "error in"=w905) -> ()  [unwired: 1 out]
      n157 = VISA Write(VISA resource name=w904, write buffer="MOV A 0\nMOV B 0\n", error in (no error)=w903) -> (VISA resource name out=w902:refnum<visa-resource-name>, error out=w901:errorcluster)  [unwired: 1 out]
    }
    frame #11 {
      n158 = VISA Write(VISA resource name=w915, write buffer="ERR?\n", error in (no error)=w914) -> (VISA resource name out=w913:refnum<visa-resource-name>, error out=w912:errorcluster)  [unwired: 1 out]
      n159 = VISA Read(VISA resource name=w913, byte count=u32 128, error in (no error)=w912) -> (VISA resource name out=w909:refnum<visa-resource-name>, read buffer=w907:string, error out=w908:errorcluster)  [unwired: 1 out]
      n160 = local write "RoughXYZErr?"(w907) -> ()
      n161 = VISA Close(VISA resource name=w909, error in (no error)=w908) -> ()  [unwired: 1 out]
    }
  }
